vi "Billard2025.vi"(5 "Open PDF":bool=TRUE, 7 "ball size":i32=13, 8 "band touch win":u32(colorbox)=6618880, 9 "band touch loose":u32(colorbox)=16711680, 10 "Create matlab score sheet":bool=TRUE, 11 "path":path=path "/Users/jammans/Downloads/T1") -> (0 "error out":errorcluster, 1 "summary":string="f:y; s:w; n:3; b:5; rb:1618; yb:1191; wb:41; ")   [LabVIEW 2025]
panel:
  out "white":cluster{i32, i32, i32}={207, 118, 118}
  out "yellow":cluster{i32, i32, i32}={193, 160, 78}
  out "red":cluster{i32, i32, i32}={508, 201, 125}
  out "Warnings C":string="All good, aucun Warning !"
  in  "line":string=".-"
  in  "error in":errorcluster
  out "PNG Picture":path=path "/Users/jammans/Downloads/T1/340.png"
  out "largeur":u32=480
  out "hauteur":u32=854
  out "dimension":u32=409920
  out "Pixmap en array":u32[](array[numeric])
  out "image":picture
  out "Path de la Pixmap":path=path "/Users/jammans/Documents/MakramFadel_RafaelaRebeiz_KevinJandri_JamilMansour/pixmap.bin"
  out "erreur C":errorcluster
  # "Coordonnées et score de chaque boules en live :"
  # "Note: Veuillez vous référer à la documentation \npour voir comment fonctionne l’encerclement \ndes rebonds  ainsi que le calcul du nombre \nde rebonds (bands touched) dans le ScoreSheet \net dans le Summary."
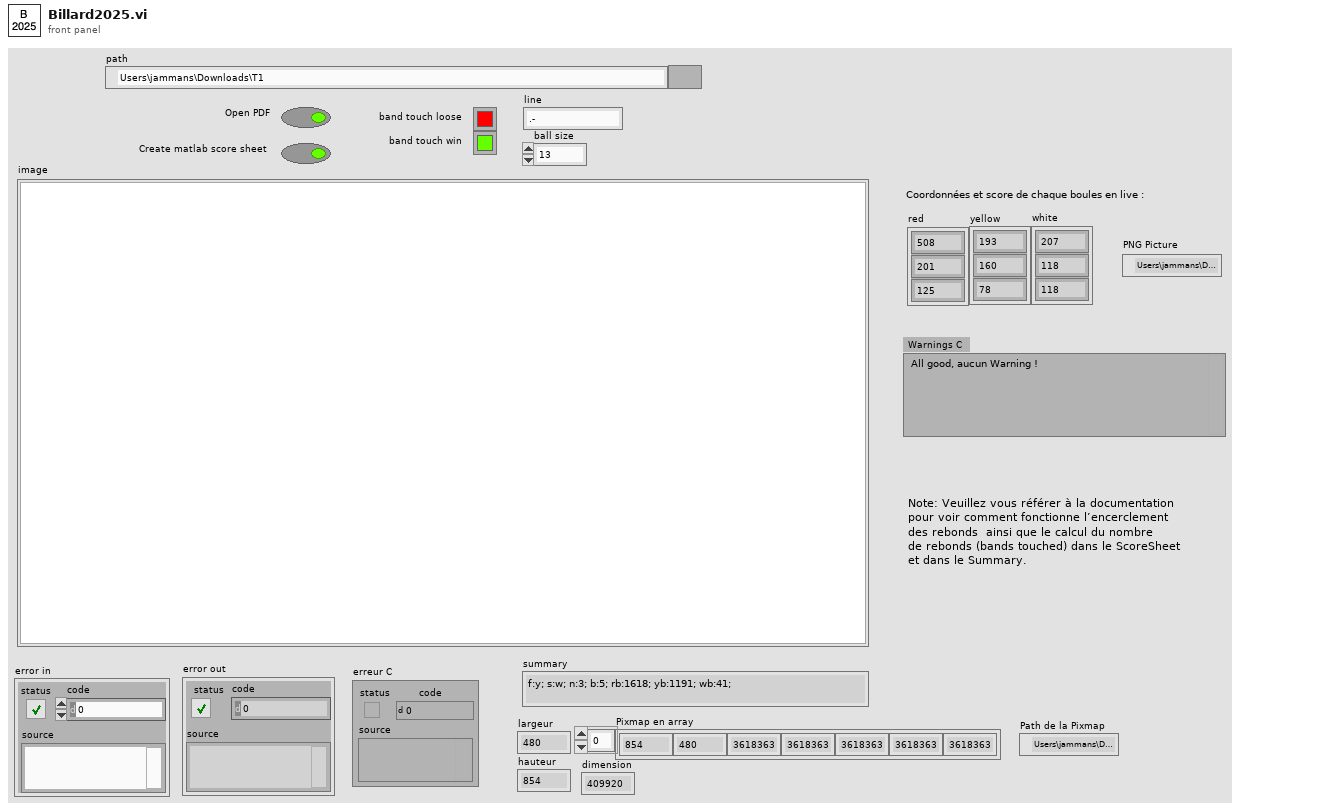
[diagram p1: front panel]
types:
  T1 = typedef "imagedata.ctl" = cluster{"image type":i32, "image depth":i32, "image":u8[], "mask":u8[], "colors":u32[], "Rectangle":cluster{"left":i16, "top":i16, "right":i16, "bottom":i16}}
  T2 = enum16{"open", "replace", "create", "open or create", "replace or create", "replace or create with confirmation"}
  T3 = enum16{"big-endian, network order", "native, host order", "little-endian"}
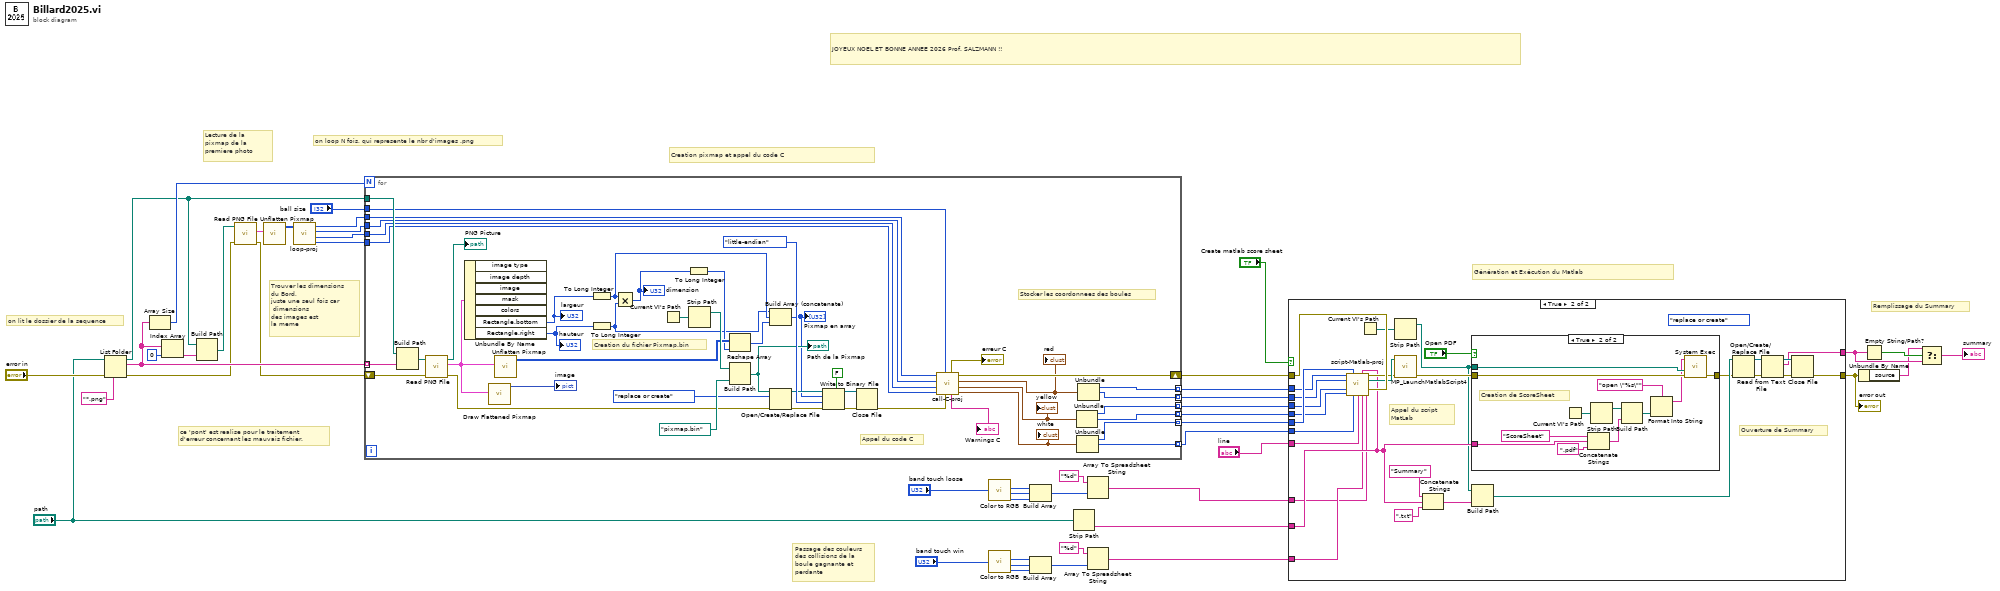
[diagram p0: block diagram]
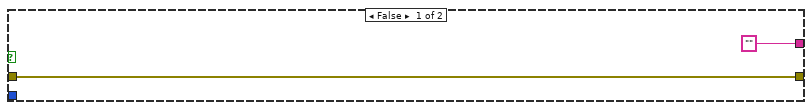
[diagram p2: hidden frame]
diagram:
  # "ce 'pont' est realise pour le traitement\nd'erreur concernant les mauvais fichier."
  # "Lecture de la pixmap de la premiere photo"
  # "Passage des couleurs des collisions de la boule gagnante et perdante"
  # "Creation pixmap et appel du code C"
  # "Génération et Exécution du Matlab"
  # "Remplissage du Summary"
  # "JOYEUX NOEL ET BONNE ANNEE 2026 Prof. SALZMANN !!"
  # "Trouver les dimensions \ndu Bord,\njuste une seul fois car\n dimensions\ndes images est \nla meme"
  # "on loop N fois, qui represente le nbr d'images .png"
  # "on lit le dossier de la sequence"
  n1 = List Folder(path="path", pattern="*.png", error in="error in") -> (path out=w32:path, filenames=w34:string[], error out=w2:errorcluster)  [unwired: 1 in, 1 out]
  n2 = Array Size(array=w34) -> (size(s)=w47:i32)
  n3 = Index Array(array=w34, index=0) -> (element=w33:string)
  n4 = Build Path(base path=w32, name or relative path=w33) -> (appended path=w31:path)
  n5 = call <vilib>:"Read PNG File.vi"("error in (no error)"=w2, "path to PNG file"=w31) -> ("error out"=w1:errorcluster, "image data"=w30:T1)  [unwired: 7 in, 1 out]
  n6 = call <vilib>:"Unflatten Pixmap.vi"("image data"=w30) -> ("24-bit pixmap"=w29:u32[][])  [unwired: 4 in, 6 out]
  n7 = call "loop-proj.vi"("pixmap"=w29) -> ("Ymax"=w25:i32, "Ymin"=w26:i32, "Xmax"=w27:i32, "Xmin"=w28:i32)  [unwired: 7 in]
  n8 = for {
    N: w47 -> [_]
    tunnel: w34 -> [w71] mode=indexing
    tunnel: w32 -> [w70]
    tunnel: [w67] -> w39 mode=indexing
    tunnel: [w66] -> w40 mode=indexing
    tunnel: [w65] -> w41 mode=indexing
    tunnel: [w64] -> w42 mode=indexing
    tunnel: [w63] -> w43 mode=indexing
    tunnel: [w62] -> w44 mode=indexing
    shift-right: [w61] -> w45
    shift-left: w1 -> [w60]
    tunnel: w28 -> [w59]
    tunnel: w27 -> [w58]
    tunnel: w26 -> [w57]
    tunnel: w25 -> [w56]
    tunnel: "ball size" -> [w55]
    # "Stocker les coordonnees des boules"
    # "Appel du code C"
    # "Creation du fichier Pixmap.bin"
    n9 = Build Path(base path=w70, name or relative path=w71) -> (appended path=w72:path)
    n10 = call <vilib>:"Read PNG File.vi"("error in (no error)"=w60, "path to PNG file"=w72) -> ("error out"=w79:errorcluster, "image data"=w92:T1, "path"=→"PNG Picture":path)  [unwired: 7 in]
    n11 = Unbundle By Name(w92) -> ("Rectangle.bottom"=w49:i16, "Rectangle.right"=w48:i16)  [unwired: 5 out]
    "largeur" <- w49
    "hauteur" <- w48
    n12 = call <vilib>:"Draw Flattened Pixmap.vi"("image data"=w92) -> ("new picture"=→"image":picture)  [unwired: 8 in]
    n13 = call <vilib>:"Unflatten Pixmap.vi"("image data"=w92) -> ("24-bit pixmap"=w85:u32[][])  [unwired: 4 in, 6 out]
    n14 = To Long Integer(number=w49) -> (32bit integer=w74:i32)
    n15 = To Long Integer(number=w48) -> (32bit integer=w73:i32)
    n16 = Multiply(x=w74, y=w73) -> (x*y=w76:i32)
    "dimension" <- w76
    n17 = Current VI's Path() -> (path=w89:path)
    n18 = To Long Integer(number=w76) -> (32bit integer=w75:i32)
    n19 = Strip Path(path=w89) -> (stripped path=w88:path)  [unwired: 1 out]
    n20 = Reshape Array(w85, w75) -> (w86:u32[])
    n21 = Build Path(base path=w88, name or relative path=path "pixmap.bin") -> (appended path=w69:path)
    "Path de la Pixmap" <- w69
    n22 = Build Array (concatenate)(w73, w74, w86) -> (w68:u32[])
    "Pixmap en array" <- w68
    n23 = Open/Create/Replace File(file path (use dialog)=w69, error in=w79, operation (0:open)=T2."replace or create") -> (refnum out=w83:refnum<file>, error out=w80:errorcluster)  [unwired: 3 in, 1 out]
    n24 = Write to Binary File(file (use dialog)=w83, data=w68, error in=w80, 5:FALSE, 9:T3."little-endian" ("byte order (0:big-endian, network order)")) -> (refnum out=w82:refnum<file>, error out=w81:errorcluster)  [unwired: 1 in, 1 out]
    n25 = Close File(refnum=w82, error in=w81) -> (error out=w78:errorcluster)  [unwired: 1 out]
    n26 = call "call-C-proj.vi"("error in"=w78, "ball size"=w55, "Ymax"=w56, "Ymin"=w57, "Xmax"=w58, "Xmin"=w59) -> ("white"=w50:cluster{i32, i32, i32}, "yellow"=w51:cluster{i32, i32, i32}, "red"=w52:cluster{i32, i32, i32}, "erreur call C"=w61:errorcluster, "Warnings C"=→"Warnings C":string, "erreur C"=→"erreur C":errorcluster)
    "red" <- w52
    "yellow" <- w51
    "white" <- w50
    n27 = Unbundle(w51) -> (w65:i32, w64:i32)  [unwired: 1 out]
    n28 = Unbundle(w50) -> (w63:i32, w62:i32)  [unwired: 1 out]
    n29 = Unbundle(w52) -> (w67:i32, w66:i32)  [unwired: 1 out]
  }
  n30 = call <vilib>:"Color to RGB.vi"("Color"="band touch loose") -> ("R"=w20:u8, "G"=w19:u8, "B"=w18:u8)  [unwired: 1 out]
  n31 = call <vilib>:"Color to RGB.vi"("Color"="band touch win") -> ("R"=w23:u8, "G"=w22:u8, "B"=w21:u8)  [unwired: 1 out]
  n32 = Build Array(w20, w19, w18) -> (w14:u8[])
  n33 = Build Array(w23, w22, w21) -> (w16:u8[])
  n34 = Strip Path(path="path") -> (name=w36:string)  [unwired: 1 out]
  n35 = Array To Spreadsheet String(array=w14, 3:"%d" ("format string")) -> (spreadsheet string=w13:string)  [unwired: 1 in]
  n36 = Array To Spreadsheet String(array=w16, 3:"%d" ("format string")) -> (spreadsheet string=w15:string)  [unwired: 1 in]
  n37 = case shown="True" "Create matlab score sheet" {
    tunnel: w45 -> [w95 w123]
    tunnel: w36 -> [_ w109]
    tunnel: w44 -> [_ w122]
    tunnel: w43 -> [_ w121]
    tunnel: w42 -> [_ w120]
    tunnel: w41 -> [_ w119]
    tunnel: w40 -> [_ w118]
    tunnel: w39 -> [_ w117]
    tunnel: w15 -> [_ w101]
    tunnel: w13 -> [_ w100]
    tunnel: [w95 w99] -> w6
    tunnel: ["" w97] -> w8
    tunnel: "line" -> [_ w96]
    frame False {
    }
    frame True {
      (unwired) T2."replace or create" ("operation (0:open)")
      # "Ouverture de Summary"
      # "Appel du script MatLab"
      n38 = call "script-Matlab-proj.vi"("Xr"=w117, "Xw"=w121, "filename"=w109, "Yr"=w118, "Xy"=w119, "error in"=w123, "Yy"=w120, "Yw"=w122, "Line"=w96, "rgb1"=w101, "rgb2"=w100) -> ("error out"=w110:errorcluster, "matlab path"=w111:path)  [unwired: 3 in]
      n39 = Current VI's Path() -> (path=w115:path)
      n40 = Strip Path(path=w115) -> (stripped path=w98:path)  [unwired: 1 out]
      n41 = call "MP_LaunchMatlabScript4.vi"("error in (no error)"=w110, "matlab script path"=w111) -> ("error out"=w108:errorcluster)  [unwired: 4 in, 5 out]
      n42 = Concatenate Strings("Summary", w109, ".txt" ("string")) -> (w113:string)
      n43 = case shown="True" "Open PDF" {
        tunnel: w109 -> [_ w131]
        tunnel: w108 -> [w124 w129]
        tunnel: [w124 w130] -> w104
        tunnel: w98 -> [_ w128]
        frame False {
        }
        frame True {
          # "Creation de ScoreSheet"
          n44 = Current VI's Path() -> (path=w136:path)
          n45 = Concatenate Strings("ScoreSheet", w131, ".pdf" ("string")) -> (w133:string)
          n46 = Strip Path(path=w136) -> (stripped path=w135:path)  [unwired: 1 out]
          n47 = Build Path(base path=w135, name or relative path=w133) -> (appended path=w127:path)
          n48 = Format Into String(format string="open \"%s\"", w127) -> (resulting string=w126:string)  [unwired: 2 in, 1 out]
          n49 = call <vilib>:"System Exec.vi"("error in (no error)"=w129, "working directory"=w128, "command line"=w126) -> ("error out"=w130:errorcluster)  [unwired: 5 in, 3 out]
        }
      }
      n50 = Build Path(base path=w98, name or relative path=w113) -> (appended path=w105:path)
      n51 = Open/Create/Replace File(file path (use dialog)=w105, error in=w104) -> (refnum out=w103:refnum<file>, error out=w102:errorcluster)  [unwired: 4 in, 1 out]
      n52 = Read from Text File(file (use dialog)=w103, error in=w102) -> (refnum out=w107:refnum<file>, text=w97:string, error out=w106:errorcluster)  [unwired: 2 in, 1 out]
      n53 = Close File(refnum=w107, error in=w106) -> (error out=w99:errorcluster)  [unwired: 1 out]
    }
  }
  "error out" <- w6
  n54 = Unbundle By Name(w6) -> ("source"=w5:string)
  n55 = Empty String/Path?(string/path=w8) -> (empty?=w9:bool)
  n56 = Select(t=w5, s=w9, f=w8) -> (s? t:f=→"summary":string)
